vi "Word Document Properties.vi"(0 "report in":refnum<class "NI_report.lvclass">, 1 "title (\"\")":string, 5 "subject (\"\")":string, 7 "author (\"\")":string, 9 "comments (\"\")":string, 11 "error in (no error)":errorcluster) -> (4 "report out":refnum<class "NI_report.lvclass">, 6 "table count":i32, 8 "shape count":i32, 15 "error out":errorcluster)   [LabVIEW 2017, in "NI_ReportGenerationToolkit.lvlib"]
doc: "Sets the properties of the current document, such as the title, subject, and author."
uses:
  <vilib>/addons/_office/NI_ReportGenerationToolkit.lvlib
  <vilib>/Utility/NIReport.llb/NI_report.lvclass
  <vilib>/Utility/NIReport.llb/Word/NI_Word.lvclass
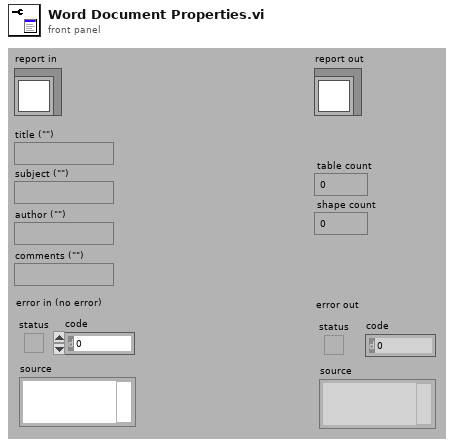
[diagram p1: front panel]
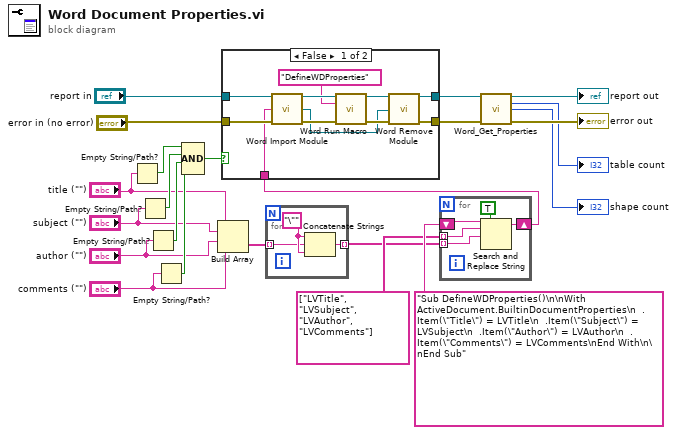
[diagram p0: block diagram]
diagram:
  n1 = Empty String/Path?(string/path="title (\"\")") -> (empty?=w20:bool)
  n2 = Empty String/Path?(string/path="subject (\"\")") -> (empty?=w19:bool)
  n3 = Empty String/Path?(string/path="author (\"\")") -> (empty?=w18:bool)
  n4 = Empty String/Path?(string/path="comments (\"\")") -> (empty?=w17:bool)
  n5 = Compound Arithmetic op=AND(w20, w19, w18, w17) -> (w16:bool)
  n6 = Build Array("title (\"\")", "subject (\"\")", "author (\"\")", "comments (\"\")") -> (w5:string[])
  n7 = for {
    tunnel: w5 -> [w24] mode=indexing
    tunnel: [w23] -> w2 mode=indexing
    w25 = "\""
    n8 = Concatenate Strings(w25, w24, w25) -> (w23:string)
  }
  n9 = for {
    shift-right: [w29] -> w1
    shift-left: "Sub DefineWDProperties()\n\nWith ActiveDocument.BuiltinDocumentProperties\n  .Item(\"Title\") = LVTitle\n  .Item(\"Subject\") = LVSubject\n  .Item(\"Author\") = LVAuthor\n  .Item(\"Comments\") = LVComments\nEnd With\n\nEnd Sub" -> [w30]
    tunnel: string[] ["LVTitle", "LVSubject", "LVAuthor", "LVComments"] ("Array Constant") -> [w27] mode=indexing
    tunnel: w2 -> [w26] mode=indexing
    n10 = Search and Replace String(replace all?=TRUE ("replace all? (F)"), input string=w30, search string=w27, replace string=w26) -> (result string=w29:string)  [unwired: 1 in, 6 out]
  }
  n11 = case shown="False" w16 {
    tunnel: "report in" -> [w35 w43]
    tunnel: "error in (no error)" -> [w34 w42]
    tunnel: [w33 w43] -> w14
    tunnel: [w32 w42] -> w15
    tunnel: w1 -> [w31 _]
    frame False {
      n12 = call <vilib>:"Word Import Module.vi"("report in"=w35, "module code (\"\")"=w31, "error in (no error)"=w34) -> ("report out"=w39:refnum<class "NI_report.lvclass">, "module reference"=w37:refnum<k7>, "error out"=w41:errorcluster)  [unwired: 1 in, 9 out]
      n13 = call <vilib>:"Word Run Macro.vi"("report in"=w39, "macro name"="DefineWDProperties", "error in (no error)"=w41) -> ("report out"=w38:refnum<class "NI_report.lvclass">, "error out"=w40:errorcluster)  [unwired: 1 in, 10 out]
      n14 = call <vilib>:"Word Remove Module.vi"("report in"=w38, "module reference"=w37, "error in (no error)"=w40) -> ("report out"=w33:refnum<class "NI_report.lvclass">, "error out"=w32:errorcluster)  [unwired: 11 out]
    }
    frame True {
    }
  }
  n15 = call <vilib>:"Word_Get_Properties.vi"("report in"=w14, "error in (no error)"=w15) -> ("report out"=→"report out":refnum<class "NI_report.lvclass">, "tables count"=→"table count":i32, "shapes count"=→"shape count":i32, "error out"=→"error out":errorcluster)  [unwired: 10 out]
